vi "Set RGB Gains.vi"(8 "Error In":errorcluster, 10 "RGB Gains":T1, 11 "Display In":refnum<class "Neopixel - RT.lvclass">) -> (0 "Error Out":errorcluster, 3 "Display Out":refnum<class "Neopixel - RT.lvclass">)   [LabVIEW 2021, in "Neopixel - RT.lvclass"]
uses:
  Neopixel - RT.lvclass
  Public/Controls/RGB Gains.ctl
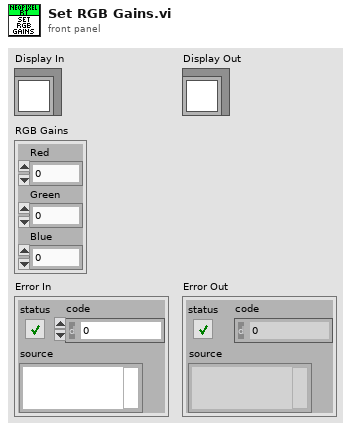
[diagram p1: front panel]
types:
  T1 = typedef "Neopixel - RT.lvclass/RGB Gains.ctl" = cluster{"Red":sgl, "Green":sgl, "Blue":sgl}
  T2 = typedef "Neopixel - RT.lvclass/Data.ctl" = cluster{"FPGA VI Reference":T3, "RGB Gains":T1}
  T3 = typedef "Neopixel - RT.lvclass/FPGA Reference.ctl" = refnum<k20>
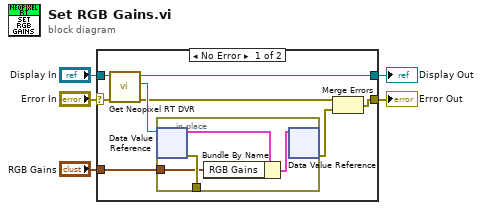
[diagram p0: block diagram]
diagram:
  n1 = case shown="No Error" "Error In" {
    selector: "Error In" -> [w9 w18]
    tunnel: [w12 w18] -> w2
    tunnel: [w7 w19] -> w3
    tunnel: "Display In" -> [w10 w19]
    tunnel: "RGB Gains" -> [w11 _]
    frame No Error {
      n2 = call "Get Neopixel RT DVR.vi"("Error In"=w9, "Display In"=w10) -> ("Error Out"=w6:errorcluster, "DVR"=w8:refnum<data-value>, "Display Out"=w7:refnum<class "Neopixel - RT.lvclass">)  [unwired: 7 in]
      n3 = in-place {
        in-place-border: [w17] -> _
        in-place-border: w11 -> [w14]
        n4 = in-place-dvr #1(w8) -> (w16:T2, w17:errorcluster)
        n5 = Bundle By Name(cluster=w16, "RGB Gains"=w14) -> (w15:T2)
        n6 = in-place-dvr #1(w15) -> (w13:errorcluster)  [unwired: 1 out]
      }
      n7 = Merge Errors(w6, w13) -> (w12:errorcluster)
    }
    frame Error {
    }
  }
  "Display Out" <- w3
  "Error Out" <- w2
